vi "errorCatcher.vi"(8 "error in (no error)":errorcluster, 11 "HWController in":refnum<class "HWController.lvclass">) -> (0 "error out":errorcluster, 3 "HWController out":refnum<class "HWController.lvclass">)   [LabVIEW 2009, in "Hardware.lvlib" / "HWControllers.lvlib" / "HWController.lvclass"]
doc: "Catch any errors that occured"
uses:
  HWController.lvclass
  HWController.lvclass/HWController.ctl
  HWControllerEvents/HWControllerEvents.lvclass
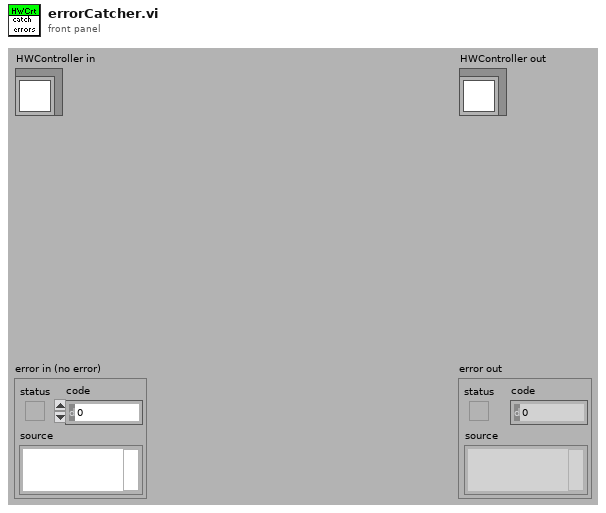
[diagram p1: front panel]
types:
  T1 = enum16{"Ready", "Compiling", "Configured", "Running", "Stopping", "Unresolved Error"}
  T2 = enum16{"start", "stop", "statusInquiry", "configure", "resetError", "resourcesInquiry", "reserveResources", "initialise", "resetAllChannels", "staticUpdate", "close", "HWStatus", "error", "resourcesAvailable", "resourcesReserved", "compilerError", "compiledScript", "compilingScript", "runScript", "configureCompiledScript"}
  T3 = cluster{"incomingEventTypes":cluster{"start":cluster{"Boolean":bool}, "stop":cluster{"Boolean":bool}, "statusInquiry":cluster{"Boolean":bool}, "configure":cluster{"DPScriptPath":path, "TimeStamp":string, "HWLoop?":bool}, "resetError":cluster{"Boolean":bool}, "resourcesInquiry":cluster{"Boolean":bool}, "reserveResources":cluster{"HWList":string[]}, "initialise":cluster{"HWList":string[]}, "close":cluster{"Boolean":bool}, "resetAllChannels":cluster{"Boolean":bool}, "staticChannelUpdate":cluster{"channel_address":string, "calibratedValue":dbl}, "runScript":cluster{"DPScriptPath":path, "TimeStamp":string, "HWLoop?":bool}, "compilingScript":cluster{"Path":path}, "compiledScript":cluster{"Path":path, "timeCompileAt":string}, "compilerError":cluster{"Path":path}, "configureCompiledScript":cluster{"DPScriptPath":path, "TimeStamp":string, "HWLoop?":bool, "CompiledScript":cluster{"ScriptListCompiler.lvclass":refnum<class "ScriptListCompiler.lvclass">, "aoChannels":refnum<class "AnalogOutput.lvclass">[], "doChannels":refnum<class "DigitalOutput.lvclass">[], "rfChannels":refnum<class "DDSOutput.lvclass">[]}}, "restartCompiler":cluster{"restart":bool}, "staticRfChannelUpdate":cluster{"channel_address":string, "Output":cluster{"Frequency(MHz)":dbl, "Amplitude":dbl, "Phase":dbl, "OutputForm":enum16{"Sine", "Square", "Triangle", "Arbitrary"}}}, "cameraUpdate":cluster{"Camera":string, "Type":string, "settings":path}}, "outgoingEventTypes":cluster{"HWStatus":cluster{"status":enum16{"Ready", "Compiling", "Configured", "Running", "Stopping", "Unresolved Error"}}, "error":cluster{"error out":errorcluster}, "resourcesAvailable":cluster{"availableHWList":string[], "reservedHWList":string[]}, "resourcesReserved":cluster{"reservedHWList":string[]}}}
  T4 = cluster{"eventId":enum16{"start", "stop", "statusInquiry", "configure", "resetError", "resourcesInquiry", "reserveResources", "initialise", "resetAllChannels", "staticUpdate", "close", "HWStatus", "error", "resourcesAvailable", "resourcesReserved", "compilerError", "compiledScript", "compilingScript", "runScript", "configureCompiledScript"}, "error":cluster{"error out":errorcluster}}
  T5 = enum16{"start", "stop", "statusInquiry", "configure", "resetError", "resourcesInquiry", "reserveResources", "initialise", "resetAllChannels", "staticUpdate", "close", "HWStatus", "error", "resourcesAvailable", "resourcesReserved", "compilerError", "compiledScript", "compilingScript", "runScript", "configureCompiledScript", "restartCompiler", "staticRfChannelUpdate", "cameraUpdate"}
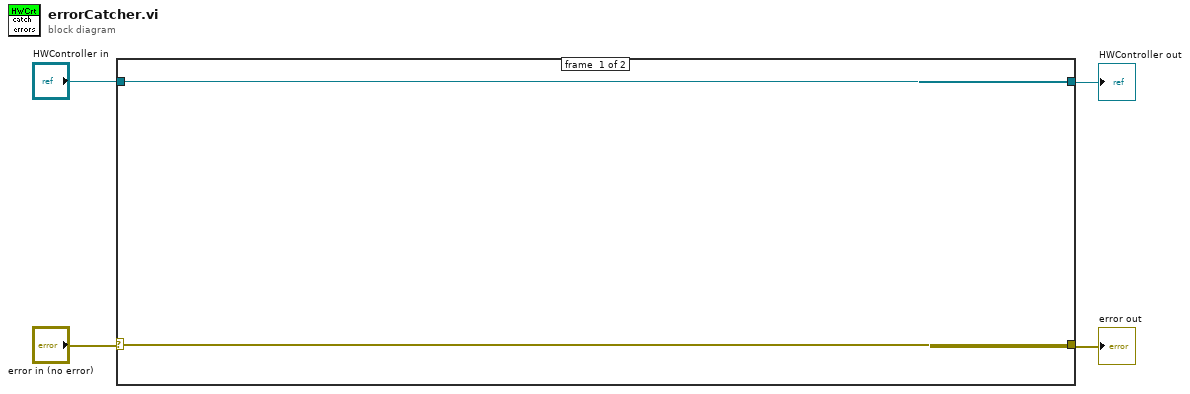
[diagram p0: block diagram]
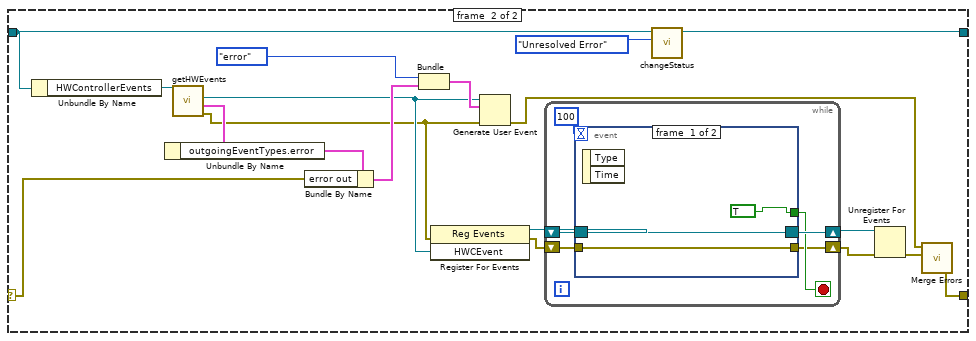
[diagram p2: hidden frame]
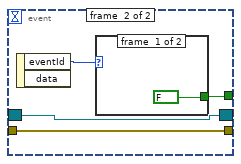
[diagram p3: hidden frame]
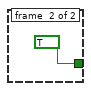
[diagram p4: hidden frame]
diagram:
  n1 = case shown="Error" "error in (no error)" {
    selector: "error in (no error)" -> [w6 w21]
    tunnel: "HWController in" -> [w5 w9]
    tunnel: [w5 w7] -> w2
    tunnel: [w6 w11] -> w1
    frame #0 {
    }
    frame #1 {
      n2 = Unbundle By Name(w9) -> ("HWControllerEvents"=w25:refnum<class "HWControllerEvents.lvclass">)
      n3 = call-dynamic "getHWEvents.vi"("HWControllerEvents in"=w25) -> ("error out"=w17:errorcluster, "eventDataTypes"=w24:T3, "HWCEvent"=w18:refnum<user-event>)  [unwired: 7 in, 1 out]
      n4 = Unbundle By Name(w24) -> ("outgoingEventTypes.error"=w22:cluster{"error out":errorcluster})
      n5 = Bundle By Name(cluster=w22, "error out"=w21) -> (w20:cluster{"error out":errorcluster})
      n6 = Bundle("eventId"=T2."error", "error"=w20) -> (w23:T4)  [unwired: 1 in]
      n7 = register-events(error in=w17, w18) -> (reference out=w19:refnum<event-registration>, error out=w16:errorcluster)  [unwired: 1 in]
      n8 = Generate User Event(user event=w18, event data cluster=w23, error in=w17) -> (error out=w13:errorcluster)  [unwired: 1 out]
      n9 = while {
        shift-right: [w30] -> w15
        shift-left: w19 -> [w31]
        shift-right: [w27] -> w14
        shift-left: w16 -> [w28]
        stop <- w29 stop-if-true
        n10 = event shown="[1] <HWCEvent>: User Event" {
          selector: w31 -> [w34 w36]
          dyn-events: [w34 w36] -> w30
          timeout: 100 -> [_ _]
          tunnel: [TRUE w37] -> w29
          tunnel: w28 -> [w32 w35]
          tunnel: [w32 w35] -> w27
          event #0 {
            n11 = event-data() -> ()  [unwired: 1 in, 2 out]
          }
          event #1 {
            n12 = event-data() -> ("eventId"=w38:T5)  [unwired: 1 in, 1 out]
            n13 = case shown="\"resetError\"" w38 {
              tunnel: [FALSE TRUE] -> w37
              frame #0 {
              }
              frame #1 {
              }
            }
          }
        }
      }
      n14 = call "changeStatus.vi"("status"=T1."Unresolved Error", "HWController in"=w9) -> ("HWController out"=w7:refnum<class "HWController.lvclass">)  [unwired: 8 in, 1 out]
      n15 = Unregister For Events(event registration refnum=w15, error in=w14) -> (error out=w12:errorcluster)
      n16 = call <vilib>:"Merge Errors.vi"("error in 2 (no error)"=w12, "error in 1 (no error)"=w13) -> ("error out"=w11:errorcluster)  [unwired: 5 in]
    }
  }
  "error out" <- w1
  "HWController out" <- w2
